vi "ClearActiveSubscription.vi"(8 "error in (no error)":errorcluster, 11 "STOMP in":refnum<class "STOMP.lvclass">) -> (0 "error out":errorcluster, 3 "STOMP out":refnum<class "STOMP.lvclass">)   [LabVIEW 2017, in "STOMP.lvclass"]
uses:
  STOMP.lvclass
  STOMP.lvclass/STOMP.ctl
  Typedefs/Type_ActiveSubscription.ctl
  Typedefs/Type_AckHeader.ctl
  Typedefs/Type_FrameHeader.ctl
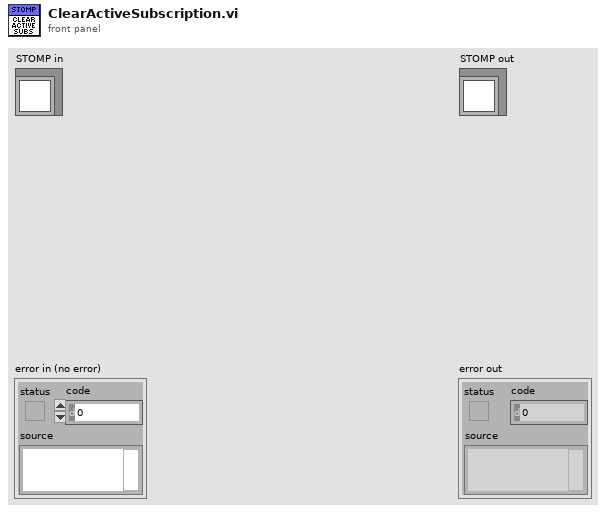
[diagram p1: front panel]
types:
  T1 = typedef "STOMP.lvclass/Type_ActiveSubscription.ctl" = cluster{"id":u64, "receipt":bool, "Destination":string, "ack":T2, "headers":T3[]}
  T2 = typedef "STOMP.lvclass/Type_AckHeader.ctl" = enum16{"auto", "client", "client-individual"}
  T3 = typedef "STOMP.lvclass/Type_FrameHeader.ctl" = cluster{"Header":string, "Value":string}
  T4 = typedef "LabVIEW STOMP.lvlib/STOMP.lvclass/ObjectAttributes.ctl" = cluster{"address":string, "port":u16, "ConnectionRef":refnum<k5>, "messageQueue":refnum<queue>, "receiptQueue":refnum<queue>, "errorQueue":refnum<queue>, "sendQueue":refnum<queue>, "currentReceiptNumber":u64, "currentSubscriptionId":u64, "closeConnection":bool, "activeSubscriptions":T5[]}
  T5 = typedef "Type_ActiveSubscription.ctl" = cluster{"id":u64, "receipt":bool, "Destination":string, "ack":T6, "headers":T7[]}
  T6 = typedef "Type_AckHeader.ctl" = enum16{"auto", "client", "client-individual"}
  T7 = typedef "LabVIEW STOMP.lvlib/STOMP.lvclass/Type_FrameHeader.ctl" = cluster{"Header":string, "Value":string}
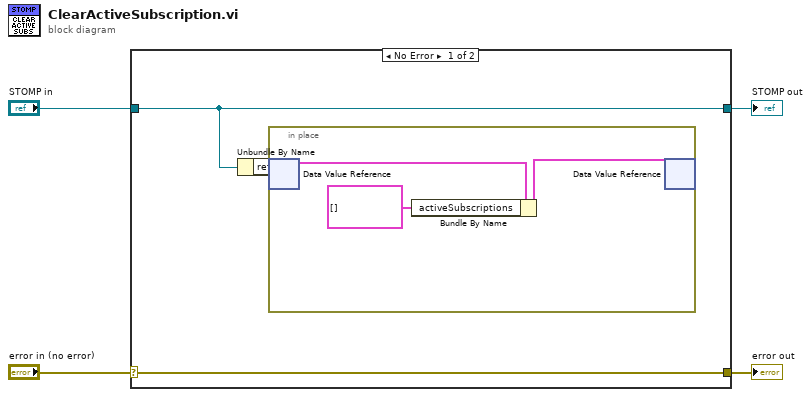
[diagram p0: block diagram]
diagram:
  n1 = case shown="No Error" "error in (no error)" {
    selector: "error in (no error)" -> [w7 w12]
    tunnel: [w7 w12] -> w3
    tunnel: [w6 w11] -> w1
    tunnel: "STOMP in" -> [w6 w11]
    frame No Error {
      n2 = Unbundle By Name(w6) -> ("ref"=w5:refnum<data-value>)
      n3 = in-place {
        n4 = in-place-dvr #1(w5) -> (w10:T4)  [unwired: 1 out]
        n5 = Bundle By Name(cluster=w10, "activeSubscriptions"=T1[] []) -> (w9:T4)
        n6 = in-place-dvr #1(w9) -> ()  [unwired: 2 out]
      }
    }
    frame Error {
    }
  }
  "error out" <- w3
  "STOMP out" <- w1
